vi "make_resultant_waveform.vi"(8 "error in (no error)":errorcluster, 11 "waveform array":waveform(dbl)[](array[waveform])) -> (0 "error out":errorcluster, 3 "inspected resultant":waveform(dbl)(graph) caption="resultant waveform")   [LabVIEW 2020]
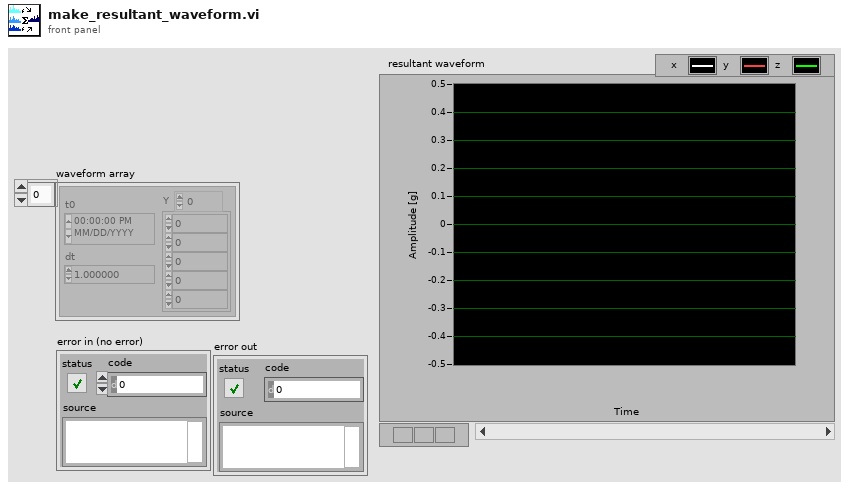
[diagram p1: front panel]
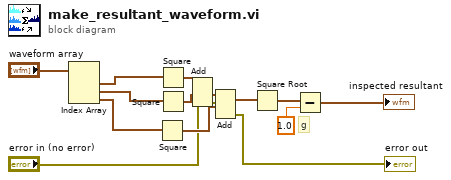
[diagram p0: block diagram]
diagram:
  # "g"
  n1 = Index Array(array="waveform array") -> (element #1=w7:waveform(dbl), element #2=w6:waveform(dbl), element #3=w5:waveform(dbl))  [unwired: 3 in]
  n2 = Square(x=w5) -> (x^2=w10:waveform(dbl))
  n3 = Square(x=w7) -> (x^2=w13:waveform(dbl))
  n4 = Square(x=w6) -> (x^2=w12:waveform(dbl))
  n5 = Add(1:w12, 2:w13, 4:"error in (no error)") -> (0:w11:waveform(dbl), 3:w3:errorcluster)
  n6 = Add(1:w10, 2:w11, 4:w3) -> (0:w9:waveform(dbl), 3:→"error out":errorcluster)
  n7 = Square Root(x=w9) -> (sqrt(x)=w14:waveform(dbl))
  n8 = Subtract(x=w14, y=1.0) -> (x-y=→"inspected resultant":waveform(dbl))
